vi "Read FF buffers.vi"(8 "error in (no error)":errorcluster, 10 "Force":bool, 11 "FpgaRef5785 in":refnum<class "FpgaRefx410.lvclass">) -> (0 "error out":errorcluster, 2 "Scaled":dbl[][](array[numeric]), 3 "FpgaRef5785 out":refnum<class "FpgaRefx410.lvclass">)   [LabVIEW 2025, in "FpgaRefx410.lvclass"]
uses:
  FpgaRefx410.lvclass
  FpgaRefx410.lvclass/FpgaRefx410.ctl
  <vilib>/rvi/interface/nirviReadWriteControl/nirviReadWriteControl.xnode
  <vilib>/rvi/interface/Simulation/niFpgaSimulationCallBeginRW.vi
  <vilib>/rvi/errors/niLvFpgaAdjustHostInterfaceError.vi
  <userlib>/_OpenG.lib/time/time.llb/openg_time.lvlib
  <vilib>/rvi/interface/nirviMethod/nirviMethod.xnode
  <vilib>/FPGAPlugInAG/Dynamic/niLvFpga_ReadFifo_Dynamic.vi
  <vilib>/rvi/errors/niLvFpgaMergeErrorWithErrorCode.vi
  x410 FPGA ref.ctl
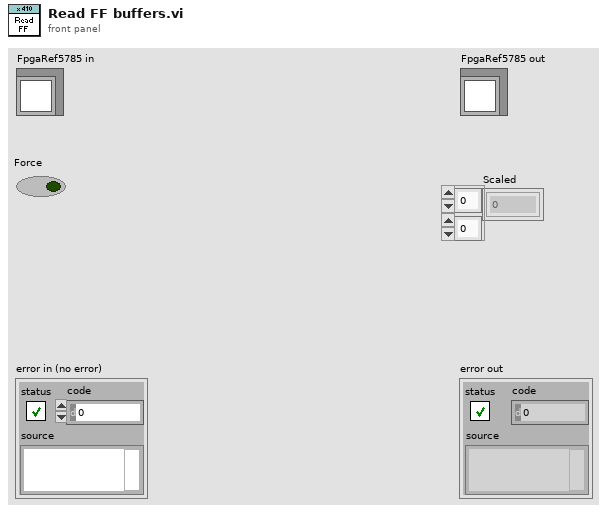
[diagram p1: front panel]
types:
  T1 = typedef "x410 FPGA ref.ctl" = refnum<k20>
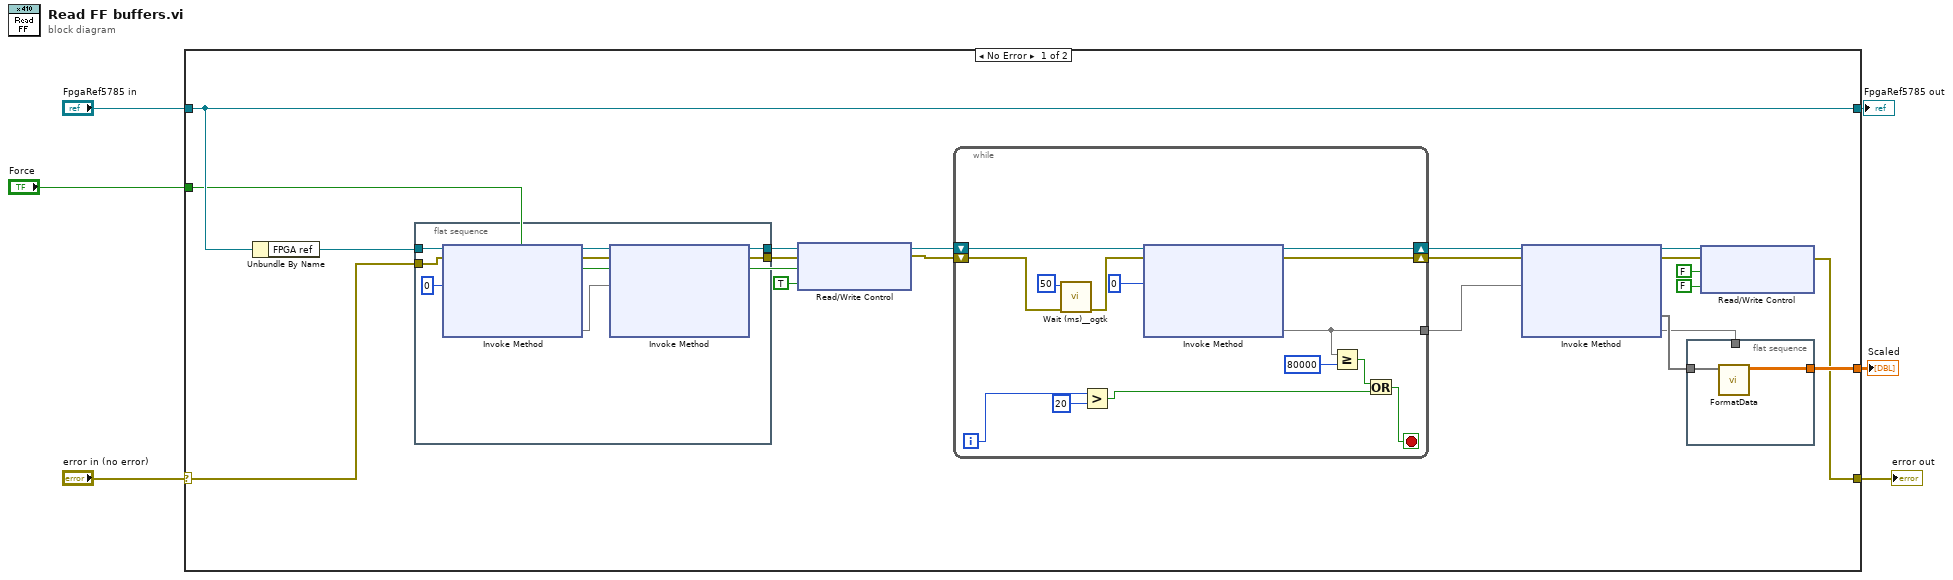
[diagram p0: block diagram]
diagram:
  n1 = case shown="No Error" "error in (no error)" {
    selector: "error in (no error)" -> [w13 w52]
    tunnel: [w12 w52] -> w5
    tunnel: [w16 w51] -> w3
    tunnel: "FpgaRef5785 in" -> [w16 w51]
    tunnel: [w14 _] -> w2
    tunnel: "Force" -> [w11 _]
    frame No Error {
      n2 = Unbundle By Name(w16) -> ("FPGA ref"=w15:T1)
      n3 = flat-sequence {
        tunnel: w15 -> [w46]
        tunnel: [w44] -> w26
        tunnel: [w42] -> w19
        tunnel: w13 -> [w41]
        frame #0 {
          n4 = xnode "Invoke Method"("FPGA VI Reference In"=w46, "error in"=w41, "Number of Elements"=u32 0) -> ("FPGA VI Reference Out"=w45:T1, "error out"=w43:errorcluster, "Elements Remaining"=w47)  [unwired: 1 in, 1 out]
          n5 = xnode "Invoke Method"("FPGA VI Reference In"=w45, "error in"=w43, "Number of Elements"=w47) -> ("FPGA VI Reference Out"=w44:T1, "error out"=w42:errorcluster)  [unwired: 1 in, 2 out]
        }
      }
      n6 = xnode "Read/Write Control"("FPGA VI Reference In"=w26, "error in"=w19, "FF buffers manual"=w11, "Load FF"=TRUE) -> ("FPGA VI Reference Out"=w7:T1, "error out"=w24:errorcluster)
      n7 = while {
        tunnel: [w27] -> w22
        shift-right: [w36] -> w18
        shift-left: w24 -> [w40]
        shift-right: [w39] -> w23
        shift-left: w7 -> [w35]
        i -> [w32]
        stop <- w28 stop-if-true
        n8 = call <userlib>:"Wait (ms)__ogtk.vi"("error in (no error)"=w40, "milliseconds to wait"=u32 50) -> ("error out"=w37:errorcluster)  [unwired: 8 in, 1 out]
        n9 = Greater?(x=w32, y=20) -> (0:w29:bool)
        n10 = xnode "Invoke Method"("FPGA VI Reference In"=w35, "error in"=w37, "Number of Elements"=u32 0) -> ("FPGA VI Reference Out"=w39:T1, "error out"=w36:errorcluster, "Elements Remaining"=w27)  [unwired: 1 in, 1 out]
        n11 = Greater Or Equal?(x=w27, y=u32 80000) -> (x >= y?=w30:bool)
        n12 = Or(x=w30, y=w29) -> (x .or. y?=w28:bool)
      }
      n13 = xnode "Invoke Method"("FPGA VI Reference In"=w23, "error in"=w18, "Number of Elements"=w22) -> ("FPGA VI Reference Out"=w20:T1, "error out"=w17:errorcluster, "Data"=w10:void[], "Elements Remaining"=w8)  [unwired: 1 in]
      n14 = flat-sequence {
        tunnel: w10 -> [w50]
        tunnel: [w49] -> w14
        tunnel: w8 -> [_]
        frame #0 {
          n15 = call "FormatData.vi"("Raw data"=w50) -> ("Scaled"=w49:dbl[][])  [unwired: 10 in]
        }
      }
      n16 = xnode "Read/Write Control"("FPGA VI Reference In"=w20, "error in"=w17, "FF buffers manual"=FALSE ("Load FF"), "Load FF"=FALSE ("FF buffers manual")) -> ("error out"=w12:errorcluster)  [unwired: 1 out]
    }
    frame Error {
    }
  }
  "error out" <- w5
  "FpgaRef5785 out" <- w3
  "Scaled" <- w2
